vi "take_snapshots_defined_voltage_profile.vi"() -> ()   [LabVIEW 2019]
uses:
  <vilib>/userDefined/High Color/IMAQdx.ctl
  <vilib>/vision/driver/IMAQdx.llb/IMAQdx Attribute Type.ctl
  <vilib>/vision/Management.llb/Cast Image 2 Method.ctl
  <vilib>/DAQmx/write.llb/DAQmx Write (Analog DBL 1Chan 1Samp).vi
  <vilib>/DAQmx/read.llb/DAQmx Read (Analog DBL 1Chan 1Samp).vi
  <vilib>/Analysis/baseanly.llb/Mean (DBL).vi
  <vilib>/DAQmx/create/channels.llb/DAQmx Create Channel (AO-Voltage-Basic).vi
  <vilib>/DAQmx/miscellaneous.llb/DAQmx Fill In Error Info.vi
  <vilib>/DAQmx/create/channels.llb/DAQmx Create Channel (AI-Temperature-Thermocouple).vi
  <vilib>/vision/driver/NI_Vision_Acquisition_Software.lvlib
  <resource>/objmgr/imaqdx.rc
  <vilib>/vision/NI_Vision_Development_Module.lvlib
  <vilib>/Analysis/NI_AALBase.lvlib
  <instrlib>/BK Precision 178XB Series/BK Precision 178XB Series.lvlib
panel:
  out "substring before match":string
  out "number":dbl
  in  "file (use dialog)":path
  in  "DC power supply":refnum<visa-resource-name>="COM3"
  in  "exit PID loop":bool
  in  "Experiment duration\n(min)":dbl
  in  "Snapshot Period\n (min per snapshot)":dbl
  out "Video":bool
  in  "Action":i32(listbox)=1
  out "meanIntensity":dbl[](array[numeric])
  out "varLaplacian":dbl[](array[numeric])
  out "mean":dbl
  out "variance":dbl
  out "Avg Intensity":dbl(graph)=4.716017316017316
  in  "Activate":bool
  out "Var of Laplacian":dbl(graph)=63.940469067936796
  in  "ROI":T1={"Global Rectangle"=[], "Contours"=[{"Contour Type"=0, "ROI Type"=3, "Points"=[231, 86, 235, 90]}, {"Contour Type"=0, "ROI Type"=3, "Points"=[193, 50, 270, 125]}]}
  in  "error in":errorcluster
  in  "File path for video":string="C:\\Users\\Aniket\\Desktop\\mCherry_calibration\\new_lens\\laser_calibration\\laser_and_heating\\"
  in  "Laser profile file path":path=path "C:/Users/Aniket/Desktop/mCherry_calibration/new_lens/laser_calibration/laser_profiles/new_profile.txt"
  in  "Trigger Laser":bool
  in  "Image file path \n(Do not add specify file extension - set to png)":path=path "C:/Users/Aniket/Desktop/mCherry_calibration/new_lens/laser_calibration/laser_profiles.txt"
  out "Current \nTemperature":dbl format="%0.2f"
  out "?":dbl[](graph)=[37.63236695538445]
  out "error out 7":errorcluster
  out "error out 6":errorcluster
  out "error out 5":errorcluster
  out "Exposure Time":dbl
  in  "ON/OFF":bool
  out "error out 3":errorcluster
  in  "LED":dbl(slide) scale=0.0..10.0
  in  "Refresh":bool
  out "Record":bool
  out "Processed Frames per Second":dbl
  out "Acquired Frame Rate":dbl
  out "error out":errorcluster
  out "Camera Display":T2(plugin-control) caption="Image Out"
  in  "Frame Rate":dbl=20.0
  out "Attribute Information Array":T4(array[cluster])
  in  "Session In":T5="cam0"
  # "Camera frame"
  # "Observer frame"
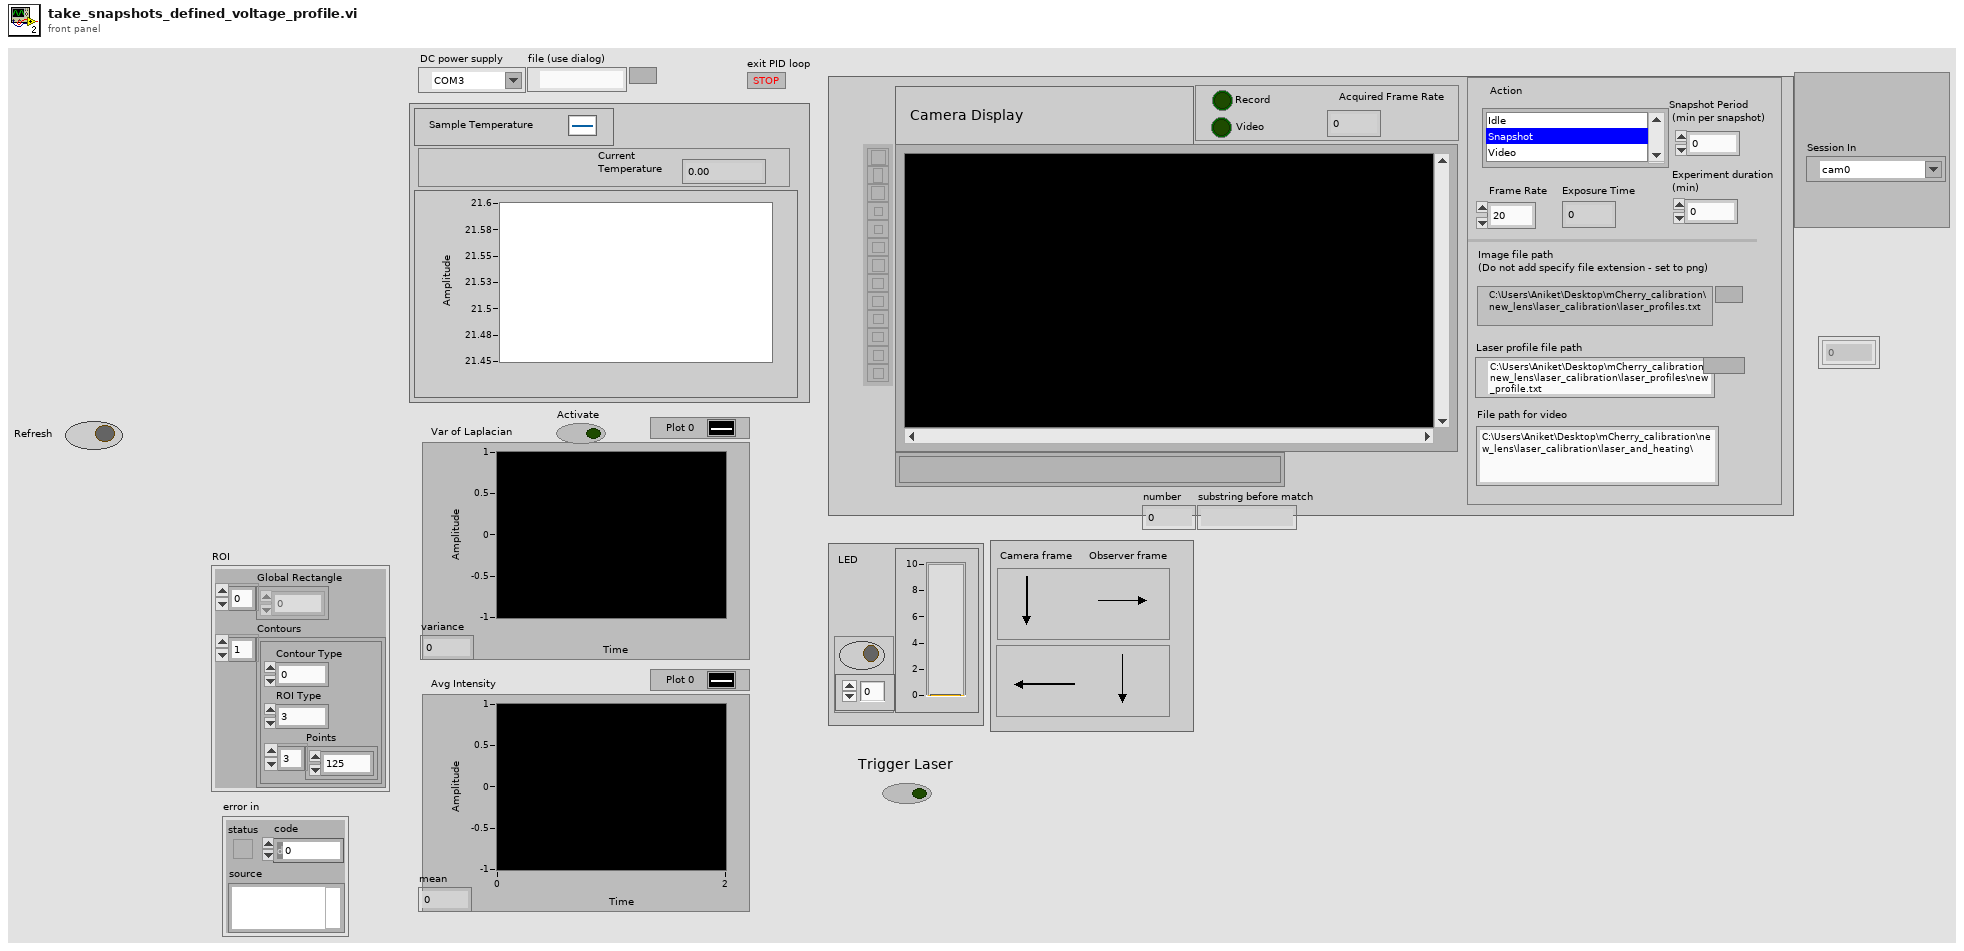
[diagram p1: front panel]
types:
  T1 = cluster{"Global Rectangle":i32[], "Contours":cluster{"Contour Type":u32, "ROI Type":u32, "Points":i32[]}[]}
  T2 = typedef "IMAQ Image.ctl" = refnum<image>
  T3 = typedef "NI_Vision_Acquisition_Software.lvlib/IMAQdx Attribute Type.ctl" = enum32{"U32", "I64", "DBL", "String", "Enum", "Bool", "Command"}
  T4 = cluster{"Attribute Type":T3, "Readable":bool, "Writable":bool, "Attribute Name":string}[]
  T5 = typedef "IMAQdx.ctl" = refnum<k21>
  T6 = typedef "Image Type" = u32
  T7 = typedef "ROI Descriptor" = cluster{"Global Rectangle":i32[], "Contours":cluster{"ID":enum32{"External", "Internal"}, "Type":u32, "Coordinates":i32[]}[]}
  T8 = typedef "IMAQ Rectangle" = cluster{"Left":i32, "Top":i32, "Right":i32, "Bottom":i32, "Rotation":dbl}
  T9 = typedef "Cast Image 2 Method.ctl" = u32
  T10 = typedef "IMAQ AVI2 Refnum.ctl" = refnum<k20>
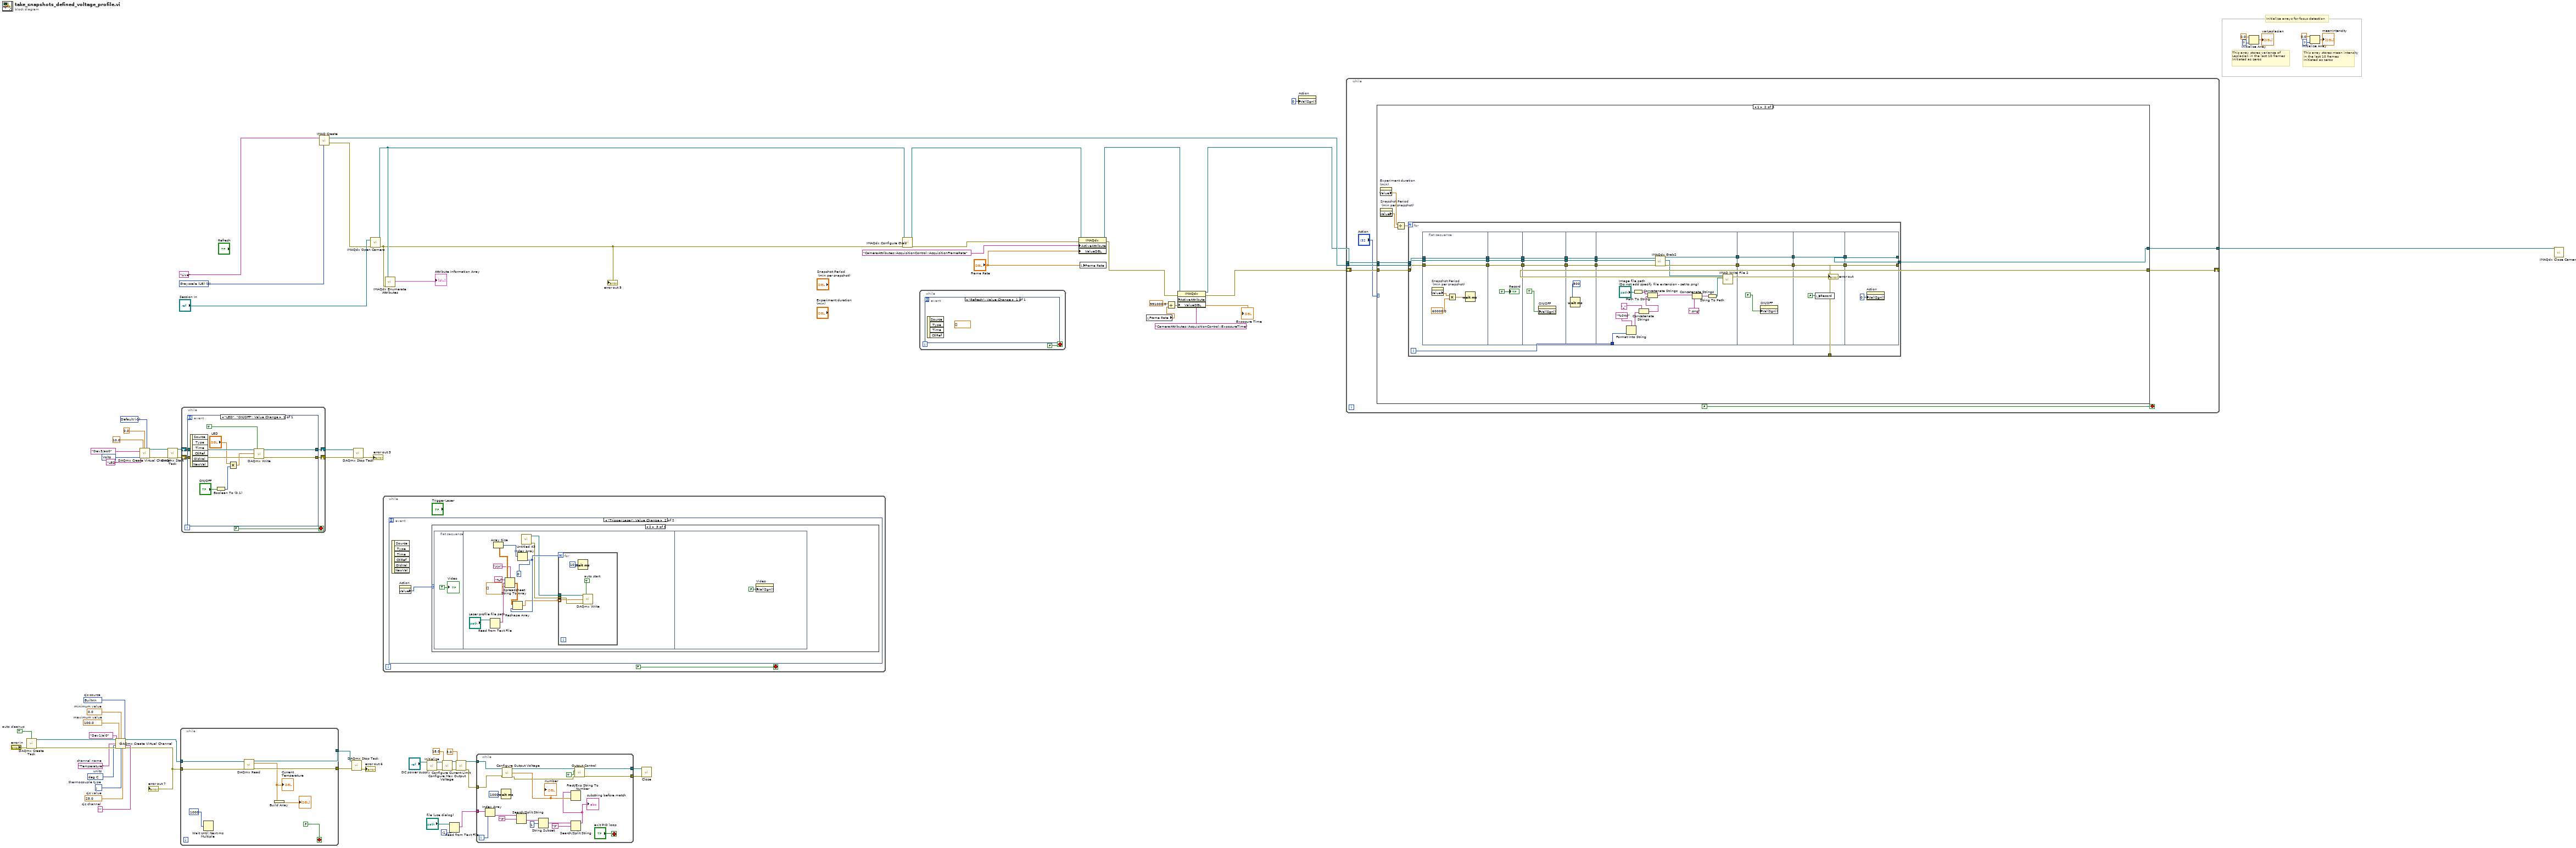
[diagram p0: block diagram]
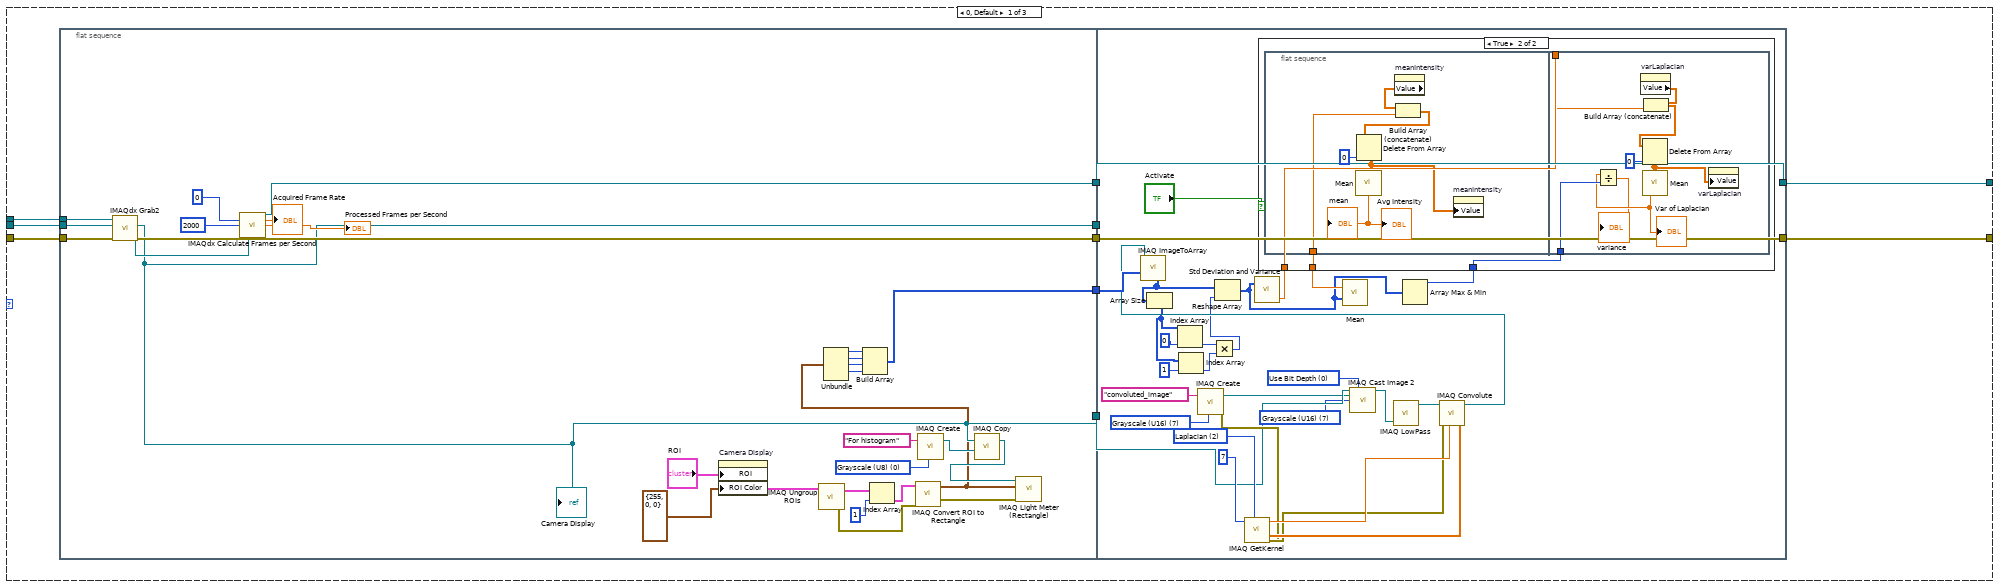
[diagram p2: hidden frame]
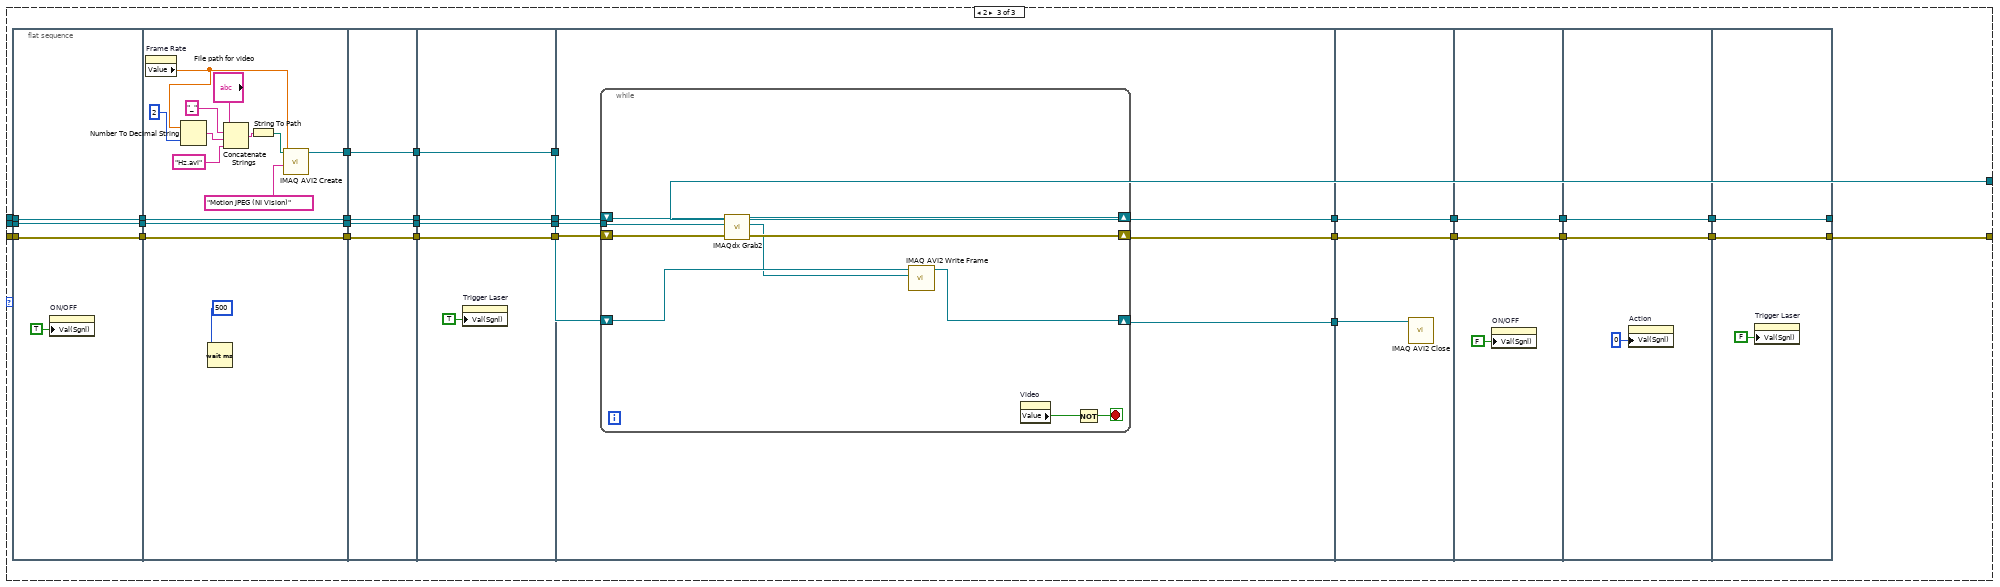
[diagram p4: hidden frame]
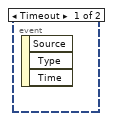
[diagram p5: hidden frame]
diagram:
  w27 = 10200 items=["Built-In"=10200, "Constant Value"=10116, "Channel"=10113]  # cjc source
  w29 = ""  # cjc channel
  w30 = 25.0  # cjc value
  w31 = 10072 items=["J"=10072, "K"=10073, "N"=10077, "R"=10082, "S"=10085, "T"=10086, "B"=10047, "E"=10055]  # thermocouple type
  w32 = 10143 items=["deg C"=10143, "deg F"=10144, "Kelvins"=10325, "deg R"=10145, "From Custom Scale"=10065]  # units
  w28 = "Temperature"  # channel name
  w33 = 0.0  # minimum value
  w34 = 100.0  # maximum value
  w36 = TRUE  # auto cleanup
  w59 = 10348 items=["Volts"=10348, "From Custom Scale"=10065] ("units")
  w61 = -1 items=["Default"=-1, "RSE"=10083, "NRSE"=10078, "Differential"=10106, "Pseudodifferential"=12529] ("input terminal configuration")
  w72 = T6 0 items=["Grayscale (U8)", "Grayscale (I16)", "Grayscale (SGL)", "Complex (CSG)", "RGB (U32)", "HSL (U32)", "RGB (U64)", "Grayscale (U16)"] ("Image Type")
  # "Initialize arrays for focus detection"
  # "This array stores mean intensity in the last 10 frames\nInitiated as zeros"
  # "This array stores variance of Laplacian in the last 10 frames\nInitiated as zeros"
  n1 = call <vilib>:"DAQmx Create Task.vi"("auto cleanup"=w36, "error in"="error in") -> ("task out"=w35:refnum<k21>, "error out"=w37:errorcluster)  [unwired: 12 in]
  n2 = call-poly <vilib>:"DAQmx Create Virtual Channel.vi"("task in"=w35, "maximum value"=w34, "minimum value"=w33, "physical channels"=tag "Dev1/ai0", "cjc source"=w27, "name to assign"=w28, "units"=w32, "cjc channel"=w29, "error in"=w37, "thermocouple type"=w31, "cjc value"=w30) -> ("task out"=w26:refnum<k21>, "error out"=w25:errorcluster)  [unwired: 3 in]
  "error out 7" <- w25
  n3 = call-poly <vilib>:"DAQmx Create Virtual Channel.vi"("maximum value"=10.0, "minimum value"=0.0, "output terminal configuration"=w61, "physical channels"=tag "Dev3/ao0", "name to assign"="LED", "units"=w59) -> ("task out"=w57:refnum<k21>, "error out"=w56:errorcluster)  [unwired: 8 in]
  n4 = call <vilib>:"DAQmx Start Task.vi"("task/channels in"=w57, "error in"=w56) -> ("task out"=w55:refnum<k21>, "error out"=w54:errorcluster)  [unwired: 12 in]
  n5 = while {
    tunnel: w26 -> [w81]
    tunnel: w25 -> [w80]
    tunnel: [w79] -> w41
    tunnel: [w78] -> w40
    stop <- FALSE ("Monitor Temperature") stop-if-true
    n6 = Wait Until Next ms Multiple(millisecond multiple=u32 1000 ("millisecond timer value")) -> ()  [unwired: 1 out]
    n7 = call-poly <vilib>:"DAQmx Read.vi"("task/channels in"=w81, "error in"=w80) -> ("task out"=w79:refnum<k21>, "data"=w75:dbl, "error out"=w78:errorcluster)  [unwired: 11 in]
    "Current \nTemperature" <- w75
    n8 = Build Array(w75) -> (→"?":dbl[])
  }
  n9 = while {
    shift-right: [w85] -> w53
    shift-left: w55 -> [w87]
    shift-right: [w84] -> w52
    shift-left: w54 -> [w86]
    stop <- FALSE stop-if-true
    n10 = event shown="[0] \"LED\", \"ON/OFF\": Value Change" {
      selector: _ -> [_]
      dyn-events: _ -> [_]
      timeout: _ -> [_]
      tunnel: w87 -> [w96]
      tunnel: w86 -> [w95]
      tunnel: [w94] -> w85
      tunnel: [w93] -> w84
      event "LED", "ON/OFF": Value Change {
        n11 = event-data() -> ()  [unwired: 1 in, 6 out]
        n12 = Boolean To (0,1)(Boolean="ON/OFF") -> (0, 1=w89:i16)
        n13 = Multiply(x="LED", y=w89) -> (x*y=w88:dbl)
        n14 = call-poly <vilib>:"DAQmx Write.vi"("task/channels in"=w96, "auto start"=TRUE, "data"=w88, "error in"=w95) -> ("task out"=w94:refnum<k21>, "error out"=w93:errorcluster)  [unwired: 9 in, 1 out]
      }
    }
  }
  n15 = call "IMAQ Create"("Image Name"="Live", "Image Type"=w72) -> ("New Image"=w66:T2, "error out"=w65:errorcluster)  [unwired: 3 in]
  n16 = call <vilib>:"DAQmx Stop Task.vi"("task/channels in"=w41, "error in"=w40) -> ("error out"=→"error out 6":errorcluster)  [unwired: 12 in, 1 out]
  n17 = call <vilib>:"DAQmx Stop Task.vi"("task/channels in"=w53, "error in"=w52) -> ("error out"=→"error out 3":errorcluster)  [unwired: 12 in, 1 out]
  n18 = call <vilib>:"IMAQdx Open Camera.vi"("error in"=w65, "Session In"="Session In") -> ("error out"=w70:errorcluster, "Session Out"=w71:T5)  [unwired: 8 in]
  "error out 5" <- w70
  n19 = while {
    stop <- FALSE stop-if-true
    n20 = event shown="[1] \"Trigger Laser\": Value Change" {
      selector: _ -> [_ _]
      dyn-events: _ -> [_ _]
      timeout: _ -> [_ _]
      event Timeout {
        n21 = event-data() -> ()  [unwired: 1 in, 3 out]
      }
      event "Trigger Laser": Value Change {
        n22 = event-data() -> ()  [unwired: 1 in, 6 out]
        n23 = property on="Action" class="LstBox (strict)"() -> ("Value"=w98:i32)  [unwired: 2 in, 2 out]
        n24 = case shown="2" w98 {
          frame 0, Default {
          }
          frame 1 {
          }
          frame 2 {
            n25 = flat-sequence {
              frame #0 {
                "Video" <- TRUE ("Video")
              }
              frame #1 {
                n26 = Read from Text File(file (use dialog)="Laser profile file path") -> (text=w107:string)  [unwired: 3 in, 3 out]
                n27 = Spreadsheet String To Array(delimiter (Tab)="\r\n", format string="%f", spreadsheet string=w107, array type (2D Dbl)=dbl[][] []) -> (array=w109:dbl[][])
                n28 = Array Size(array=w109) -> (size(s)=w108:i32[])
                n29 = Index Array(array=w108, index=0) -> (element=w111:i32)
                n30 = Reshape Array(w109, w111) -> (w110:dbl[])
                n31 = call "Untitled 43.vi"() -> ("error out"=w100:errorcluster, "task out"=w101:refnum<k21>)  [unwired: 10 in]
                n32 = for {
                  N: w111 -> [_]
                  tunnel: w110 -> [w112] mode=indexing
                  tunnel: w101 -> [w114]
                  tunnel: w100 -> [w113]
                  w115 = TRUE  # auto start
                  n33 = Wait (ms)(milliseconds to wait=u32 10) -> ()  [unwired: 1 out]
                  n34 = call-poly <vilib>:"DAQmx Write.vi"("task/channels in"=w114, "auto start"=w115, "data"=w112, "error in"=w113) -> ()  [unwired: 9 in, 3 out]
                }
              }
              frame #2 {
                n35 = property on="Video" class="Bool (strict)"("Val(Sgnl)"=FALSE ("Value (Signaling)")) -> ()  [unwired: 2 in, 2 out]
              }
            }
          }
        }
      }
    }
  }
  n36 = call <vilib>:"IMAQdx Enumerate Attributes.vi"("error in"=w70, "Session In"=w71) -> ("Attribute Information Array"=→"Attribute Information Array":T4)  [unwired: 7 in, 2 out]
  n37 = call "Initialize.vi"("VISA resource name"="DC power supply") -> ("error out"=w11:errorcluster, "VISA resource name out"=w13:refnum<visa-resource-name>)  [unwired: 9 in]
  n38 = call "Configure Max Output Voltage.vi"("VISA resource name"=w13, "Maximum Output Voltage (18)"=18.0, "error in (no error)"=w11) -> ("VISA resource name out"=w12:refnum<visa-resource-name>, "error out"=w10:errorcluster)  [unwired: 11 in]
  n39 = Read from Text File(file (use dialog)="file (use dialog)", count=-1) -> (text=w7:string[])  [unwired: 2 in, 3 out]
  n40 = call "Configure Current Limit.vi"("VISA resource name"=w12, "Current Limit (0)"=3.0, "error in (no error)"=w10) -> ("VISA resource name out"=w4:refnum<visa-resource-name>, "error out"=w5:errorcluster)  [unwired: 11 in]
  n41 = while {
    tunnel: w7 -> [w135]
    tunnel: [w121] -> w6
    tunnel: w5 -> [w123]
    tunnel: w4 -> [w124]
    tunnel: [w118] -> w3
    i -> [w134]
    stop <- "exit PID loop" stop-if-true
    n42 = Index Array(array=w135, index=w134) -> (element=w133:string)
    n43 = Wait (ms)(milliseconds to wait=u32 1000) -> ()  [unwired: 1 out]
    n44 = Search/Split String(string=w133, search string/char (-)="\t") -> (match + rest of string=w128:string)  [unwired: 1 in, 2 out]
    n45 = String Subset(string=w128, offset (0)=1) -> (substring=w129:string)  [unwired: 1 in]
    n46 = Search/Split String(string=w129, search string/char (-)="\t") -> (substring before match=w126:string)  [unwired: 1 in, 2 out]
    "substring before match" <- w126
    n47 = Fract/Exp String To Number(string=w126) -> (number=w127:dbl)  [unwired: 3 in, 1 out]
    "number" <- w127
    n48 = call "Configure Output Voltage.vi"("VISA resource name"=w124, "Output Voltage (0)"=w127, "error in (no error)"=w123) -> ("VISA resource name out"=w122:refnum<visa-resource-name>, "error out"=w119:errorcluster)  [unwired: 11 in]
    n49 = call "Output Control.vi"("error in (no error)"=w119, "Enable Output Terminals (F: Off)"=TRUE, "VISA resource name"=w122) -> ("error out"=w118:errorcluster, "VISA resource name out"=w121:refnum<visa-resource-name>)  [unwired: 7 in]
  }
  n50 = call "Close.vi"("error in (no error)"=w3, "VISA resource name"=w6) -> ()  [unwired: 9 in, 1 out]
  n51 = call <vilib>:"IMAQdx Configure Grab.vi"("error in"=w70, "Session In"=w71) -> ("error out"=w68:errorcluster, "Session Out"=w50:T5)  [unwired: 8 in]
  n52 = while {
    stop <- FALSE stop-if-true
    n53 = event shown="[0] \"Refresh\": Value Change" {
      selector: _ -> [_]
      dyn-events: _ -> [_]
      timeout: _ -> [_]
      event "Refresh": Value Change {
        (unwired) dbl[] [] ("History Data")
        n54 = event-data() -> ()  [unwired: 1 in, 4 out]
      }
    }
  }
  n55 = property class="IMAQdx"(reference=w50, error in=w68, "ActiveAttribute"="CameraAttributes::AcquisitionControl::AcquisitionFrameRate", "ValueDBL"="Frame Rate") -> (reference out=w45:T5, error out=w43:errorcluster)
  n56 = local write "Frame Rate"("Frame Rate") -> ()
  n57 = local read "Frame Rate"() -> (w47:dbl)
  n58 = Divide(x=991000.0, y=w47) -> (x/y=w46:dbl)
  "Exposure Time" <- w46
  n59 = property class="IMAQdx"(reference=w45, error in=w43, "ActiveAttribute"="CameraAttributes::AcquisitionControl::ExposureTime", "ValueDBL"=w46) -> (reference out=w44:T5, error out=w42:errorcluster)
  n60 = property on="Action" class="LstBox (strict)"("Val(Sgnl)"=0 ("Value (Signaling)")) -> ()  [unwired: 2 in, 2 out]
  n61 = while {
    tunnel: w44 -> [w144]
    tunnel: w66 -> [w142]
    shift-right: [w141] -> w15
    shift-left: w42 -> [w143]
    tunnel: [w138] -> w17
    stop <- FALSE ("Stop") stop-if-true
    n62 = case shown="1" "Action" {
      tunnel: w144 -> [w154 w237 w334]
      tunnel: w143 -> [w153 w235 w332]
      tunnel: w142 -> [w152 w236 w333]
      tunnel: [w151 w234 w330] -> w141
      tunnel: [w150 w233 w331] -> w138
      frame 0, Default {
        n63 = flat-sequence {
          tunnel: w154 -> [w182]
          tunnel: w153 -> [w181]
          tunnel: w152 -> [w180]
          tunnel: [w179] -> w149
          tunnel: [w177] -> w148
          tunnel: [w164] -> w147
          tunnel: [w164] -> w146
          tunnel: [w156] -> w145
          tunnel: [w211] -> w150
          tunnel: [w212] -> w151
          tunnel: w149 -> [w212]
          tunnel: w148 -> [w211]
          tunnel: w147 -> [_]
          tunnel: w146 -> [w192]
          tunnel: w145 -> [w202]
          frame #0 {
            w165 = T6 0 items=["Grayscale (U8)", "Grayscale (I16)", "Grayscale (SGL)", "Complex (CSG)", "RGB (U32)", "HSL (U32)", "RGB (U64)", "Grayscale (U16)"] ("Image Type")
            n64 = call <vilib>:"IMAQdx Grab2.vi"("error in"=w181, "Image In"=w180, "Session In"=w182) -> ("error out"=w179:errorcluster, "Image Out"=w164:T2, "Session Out"=w178:T5)  [unwired: 5 in, 1 out]
            "Camera Display" <- w164
            n65 = call <vilib>:"IMAQdx Calculate Frames per Second.vi"("Session In"=w178, "Buffer Number"=u32 0, "Minimum Display Update Interval (ms)"=u32 2000) -> ("Session Out"=w177:T5, "Acquired Frames per Second"=→"Acquired Frame Rate":dbl, "Processed Frames per Second"=→"Processed Frames per Second":dbl)  [unwired: 6 in, 4 out]
            n66 = property on="Camera Display" class="ImageControl"("ROI"="ROI", "ROI Color"=cluster{"Red":u8, "Green":u8, "Blue":u8} {"Red"=255, "Green"=0, "Blue"=0}) -> ()  [unwired: 2 in, 2 out]
            n67 = call "IMAQ Ungroup ROIs"("ROI Descriptor"="ROI") -> ("error out"=w168:errorcluster, "ROI Descriptors out"=w171:T7[])  [unwired: 3 in]
            n68 = Index Array(array=w171, index=1) -> (element=w169:T7)
            n69 = call "IMAQ Convert ROI to Rectangle"("error in (no error)"=w168, "ROI Descriptor"=w169) -> ("error out"=w167:errorcluster, "Rectangle"=w161:T8)  [unwired: 7 in]
            n70 = Unbundle(w161) -> ("Left"=w160:i32, "Top"=w159:i32, "Right"=w158:i32, "Bottom"=w157:i32)  [unwired: 1 out]
            n71 = Build Array(w160, w159, w158, w157) -> (w156:i32[])
            n72 = call "IMAQ Create"("Image Name"="For histogram", "Image Type"=w165) -> ("New Image"=w163:T2)  [unwired: 3 in, 1 out]
            n73 = call "IMAQ Copy"("Image Dst"=w163, "Image Src"=w164) -> ("Image Dst Out"=w162:T2)  [unwired: 4 in, 1 out]
            n74 = call "IMAQ Light Meter (Rectangle)"("error in (no error)"=w167, "Rectangle"=w161, "Image"=w162) -> ()  [unwired: 4 in, 5 out]
          }
          frame #1 {
            w188 = T6 7 items=["Grayscale (U8)", "Grayscale (I16)", "Grayscale (SGL)", "Complex (CSG)", "RGB (U32)", "HSL (U32)", "RGB (U64)", "Grayscale (U16)"] ("Image Type")
            w191 = T9 0 items=["Use Bit Depth", "Shift", "Use Lookup Table"] ("Method")
            w207 = u16 2 items=["Gradient"=1, "Laplacian"=2, "Smoothing"=3, "Gaussian"=4] ("Kernel Family")
            w209 = T6 7 items=["Grayscale (U8)", "Grayscale (I16)", "Grayscale (SGL)", "Complex (CSG)", "RGB (U32)", "HSL (U32)", "RGB (U64)", "Grayscale (U16)"] ("Image Type")
            n75 = call "IMAQ Create"("Image Name"="convoluted_image", "Image Type"=w209) -> ("New Image"=w190:T2, "error out"=w203:errorcluster)  [unwired: 3 in]
            n76 = call "IMAQ GetKernel"("Kernel Family"=w207, "error in (no error)"=w203, "Kernel Size (3,5,...)"=7) -> ("error out"=w204:errorcluster, "Kernel"=w205:sgl[][], "Divider"=w206:sgl)  [unwired: 5 in, 1 out]
            n77 = call "IMAQ Cast Image 2"("Image Src"=w192, "Method"=w191, "Image Dst"=w190, "Image Type"=w188) -> ("Image Dst Out"=w189:T2)  [unwired: 10 in, 1 out]
            n78 = call "IMAQ LowPass"("Image Src"=w189) -> ("Image Dst Out"=w193:T2)  [unwired: 6 in, 1 out]
            n79 = call "IMAQ Convolute"("Kernel"=w205, "Divider (kernel sum)"=w206, "error in (no error)"=w204, "Image Src"=w193) -> ("Image Dst Out"=w201:T2)  [unwired: 6 in, 1 out]
            n80 = call "IMAQ ImageToArray"("Optional Rectangle"=w202, "Image"=w201) -> ("Image Pixels (U16)"=w186:u16[][])  [unwired: 2 in, 4 out]
            n81 = Array Size(array=w186) -> (size(s)=w187:i32[])
            n82 = Index Array(array=w187, index=0 ("index (row)")) -> (element=w198:i32)
            n83 = Index Array(array=w187, index=1) -> (element=w197:i32)
            n84 = Multiply(x=w198, y=w197) -> (x*y=w185:i32)
            n85 = Reshape Array(w186, w185) -> (w184:u16[])
            n86 = call <vilib>:"Std Deviation and Variance.vi"("X"=w184) -> ("variance"=w195:dbl)  [unwired: 1 in, 2 out]
            n87 = call-poly <vilib>:"Mean.vi"("X"=w184) -> ("mean"=w194:dbl)  [unwired: 1 out]
            n88 = Array Max & Min(array=w184) -> (max value=w183:u16)  [unwired: 3 out]
            n89 = case shown="True" "Activate" {
              tunnel: w195 -> [_ w214]
              tunnel: w194 -> [_ w215]
              tunnel: w183 -> [_ w213]
              frame False {
              }
              frame True {
                n90 = flat-sequence {
                  tunnel: w215 -> [w218]
                  tunnel: w214 -> [w224]
                  tunnel: w213 -> [w229]
                  frame #0 {
                    n91 = property on="meanIntensity" class="Arr (strict)"() -> ("Value"=w219:dbl[])  [unwired: 2 in, 2 out]
                    n92 = Build Array (concatenate)(w219, w218) -> (w217:dbl[])
                    n93 = Delete From Array(array=w217, index=0) -> (array with subset deleted=w216:dbl[])  [unwired: 1 in, 1 out]
                    n94 = call-poly <vilib>:"Mean.vi"("X"=w216) -> ("mean"=→"Avg Intensity" →"mean":dbl)  [unwired: 1 out]
                    n95 = property on="meanIntensity" class="Arr (strict)"("Value"=w216) -> ()  [unwired: 2 in, 2 out]
                  }
                  frame #1 {
                    n96 = property on="varLaplacian" class="Arr (strict)"() -> ("Value"=w225:dbl[])  [unwired: 2 in, 2 out]
                    n97 = Build Array (concatenate)(w225, w224) -> (w223:dbl[])
                    n98 = Delete From Array(array=w223, index=0) -> (array with subset deleted=w222:dbl[])  [unwired: 1 in, 1 out]
                    n99 = call-poly <vilib>:"Mean.vi"("X"=w222) -> ("mean"=w228:dbl)  [unwired: 1 out]
                    "Var of Laplacian" <- w228
                    n100 = Divide(x=w228, y=w229) -> (x/y=→"variance":dbl)
                    n101 = property on="varLaplacian" class="Arr (strict)"("Value"=w222) -> ()  [unwired: 2 in, 2 out]
                  }
                }
              }
            }
          }
        }
      }
      frame 1 {
        n102 = property on="Experiment duration\n(min)" class="DigNum (strict)"() -> ("Value"=w231:dbl)  [unwired: 2 in, 2 out]
        n103 = property on="Snapshot Period\n (min per snapshot)" class="DigNum (strict)"() -> ("Value"=w230:dbl)  [unwired: 2 in, 2 out]
        n104 = Divide(x=w231, y=w230) -> (x/y=w232:dbl)
        n105 = for {
          N: w232 -> [_]
          tunnel: w237 -> [w246]
          tunnel: w236 -> [w245]
          tunnel: w235 -> [w244]
          tunnel: [w243] -> w234
          tunnel: [w242] -> w233
          i -> [w241]
          n106 = flat-sequence {
            tunnel: w246 -> [w265]
            tunnel: w245 -> [w266]
            tunnel: w244 -> [w267]
            tunnel: [w267] -> w240
            tunnel: [w266] -> w239
            tunnel: [w265] -> w238
            tunnel: [w271] -> w261
            tunnel: [w270] -> w260
            tunnel: [w269] -> w259
            tunnel: w238 -> [w269]
            tunnel: w239 -> [w270]
            tunnel: w240 -> [w271]
            tunnel: [w275] -> w258
            tunnel: [w274] -> w257
            tunnel: [w273] -> w256
            tunnel: w261 -> [w275]
            tunnel: w260 -> [w274]
            tunnel: w259 -> [w273]
            tunnel: w258 -> [w279]
            tunnel: [w279] -> w255
            tunnel: w257 -> [w278]
            tunnel: [w278] -> w254
            tunnel: w256 -> [w277]
            tunnel: [w277] -> w253
            tunnel: [w292] -> w252
            tunnel: [w296] -> w251
            tunnel: w255 -> [w295]
            tunnel: w254 -> [w294]
            tunnel: w253 -> [w293]
            tunnel: w241 -> [w280]
            tunnel: w252 -> [w299]
            tunnel: [w299] -> w250
            tunnel: w251 -> [w298]
            tunnel: [w298] -> w249
            tunnel: w250 -> [w302]
            tunnel: w249 -> [w301]
            tunnel: [w302] -> w248
            tunnel: [w301] -> w247
            tunnel: [w305] -> w243
            tunnel: [w303] -> w242
            tunnel: w248 -> [w303]
            tunnel: w247 -> [w305]
            frame #0 {
              n107 = property on="Snapshot Period\n (min per snapshot)" class="DigNum (strict)"() -> ("Value"=w264:dbl)  [unwired: 2 in, 2 out]
              n108 = Multiply(x=w264, y=60000.0) -> (x*y=w262:dbl)
              n109 = Wait (ms)(milliseconds to wait=w262) -> ()  [unwired: 1 out]
            }
            frame #1 {
              "Record" <- TRUE ("Record")
            }
            frame #2 {
              n110 = property on="ON/OFF" class="Bool (strict)"("Val(Sgnl)"=TRUE ("ON/OFF")) -> ()  [unwired: 2 in, 2 out]
            }
            frame #3 {
              n111 = Wait (ms)(milliseconds to wait=u32 500) -> ()  [unwired: 1 out]
            }
            frame #4 {
              n112 = Format Into String(format string="%04d", w280) -> (resulting string=w281:string)  [unwired: 2 in, 1 out]
              n113 = Path To String(path="Image file path \n(Do not add specify file extension - set to png)") -> (string=w288:string)
              n114 = Concatenate Strings("_" ("string"), w281) -> (w287:string)
              n115 = Concatenate Strings(w288, w287) -> (w286:string)
              n116 = call <vilib>:"IMAQdx Grab2.vi"("error in"=w295, "Image In"=w294, "Session In"=w293) -> ("error out"=w296:errorcluster, "Image Out"=w291:T2, "Session Out"=w292:T5)  [unwired: 5 in, 1 out]
              n117 = Concatenate Strings(w286, ".png" ("string")) -> (w284:string)
              n118 = String To Path(string=w284) -> (path=w283:path)
              n119 = call-poly "IMAQ Write File 2"("File Path"=w283, "Image"=w291) -> ()  [unwired: 8 in, 2 out]
            }
            frame #5 {
              n120 = property on="ON/OFF" class="Bool (strict)"("Val(Sgnl)"=FALSE ("ON/OFF")) -> ()  [unwired: 2 in, 2 out]
            }
            frame #6 {
              n121 = local write "Record"(FALSE ("Record")) -> ()
            }
            frame #7 {
              n122 = property on="Action" class="LstBox (strict)"("Val(Sgnl)"=0 ("Value (Signaling)")) -> ()  [unwired: 2 in, 2 out]
            }
          }
        }
      }
      frame 2 {
        n123 = flat-sequence {
          tunnel: w332 -> [w336]
          tunnel: w333 -> [w337]
          tunnel: w334 -> [w338]
          tunnel: [w338] -> w329
          tunnel: [w337] -> w328
          tunnel: [w336] -> w327
          tunnel: w329 -> [w352]
          tunnel: [w352] -> w326
          tunnel: w328 -> [w351]
          tunnel: [w351] -> w324
          tunnel: w327 -> [w350]
          tunnel: [w350] -> w322
          tunnel: [w347] -> w315
          tunnel: w326 -> [w356]
          tunnel: [w356] -> w325
          tunnel: w324 -> [w355]
          tunnel: [w355] -> w323
          tunnel: w322 -> [w354]
          tunnel: [w354] -> w321
          tunnel: [w353] -> w316
          tunnel: w315 -> [w353]
          tunnel: w325 -> [w358]
          tunnel: w323 -> [w359]
          tunnel: w321 -> [w360]
          tunnel: [w360] -> w320
          tunnel: [w359] -> w319
          tunnel: [w358] -> w318
          tunnel: [w357] -> w317
          tunnel: w316 -> [w357]
          tunnel: w320 -> [w367]
          tunnel: w319 -> [w366]
          tunnel: w318 -> [w365]
          tunnel: [w363] -> w314
          tunnel: [w364] -> w313
          tunnel: [w368] -> w312
          tunnel: w317 -> [w362]
          tunnel: w314 -> [w381]
          tunnel: [w381] -> w309
          tunnel: w313 -> [w380]
          tunnel: [w380] -> w311
          tunnel: w312 -> [w379]
          tunnel: w311 -> [w384]
          tunnel: [w384] -> w310
          tunnel: w309 -> [w383]
          tunnel: [w383] -> w308
          tunnel: w310 -> [w386]
          tunnel: w308 -> [w387]
          tunnel: [w387] -> w307
          tunnel: [w386] -> w306
          tunnel: [w389] -> w330
          tunnel: [w390] -> w331
          tunnel: w307 -> [w390]
          tunnel: w306 -> [w389]
          frame #0 {
            n124 = property on="ON/OFF" class="Bool (strict)"("Val(Sgnl)"=TRUE ("Value (Signaling)")) -> ()  [unwired: 2 in, 2 out]
          }
          frame #1 {
            n125 = property on="Frame Rate" class="DigNum (strict)"() -> ("Value"=w345:dbl)  [unwired: 2 in, 2 out]
            n126 = Number To Decimal String(number=w345, width (-)=i16 2) -> (decimal integer string=w340:string)
            n127 = Wait (ms)(milliseconds to wait=u32 500) -> ()  [unwired: 1 out]
            n128 = Concatenate Strings("File path for video", "_" ("string"), w340, "Hz.avi" ("string")) -> (w342:string)
            n129 = String To Path(string=w342) -> (path=w343:path)
            n130 = call "IMAQ AVI2 Create"("Codec"="Motion JPEG (NI Vision)", "Frames Per Second"=w345, "AVI Path"=w343) -> ("AVI Refnum"=w347:T10)  [unwired: 7 in, 1 out]
          }
          frame #2 {
          }
          frame #3 {
            n131 = property on="Trigger Laser" class="Bool (strict)"("Val(Sgnl)"=TRUE ("Value (Signaling)")) -> ()  [unwired: 2 in, 2 out]
          }
          frame #4 {
            n132 = while {
              tunnel: w366 -> [w376]
              shift-right: [w374] -> w364
              shift-left: w367 -> [w377]
              shift-right: [w373] -> w363
              shift-left: w365 -> [w375]
              shift-right: [w378] -> w368
              shift-left: w362 -> [w372]
              stop <- w370 stop-if-true
              n133 = call <vilib>:"IMAQdx Grab2.vi"("error in"=w377, "Image In"=w376, "Session In"=w375) -> ("error out"=w374:errorcluster, "Image Out"=w371:T2, "Session Out"=w373:T5)  [unwired: 5 in, 1 out]
              n134 = call "IMAQ AVI2 Write Frame"("Image"=w371, "AVI Refnum"=w372) -> ("AVI Refnum (duplicate)"=w378:T10)  [unwired: 7 in, 2 out]
              n135 = property on="Video" class="Bool (strict)"() -> ("Value"=w369:bool)  [unwired: 2 in, 2 out]
              n136 = Not(x=w369) -> (.not. x?=w370:bool)
            }
          }
          frame #5 {
            n137 = call "IMAQ AVI2 Close"("AVI Refnum"=w379) -> ()  [unwired: 10 in, 1 out]
          }
          frame #6 {
            n138 = property on="ON/OFF" class="Bool (strict)"("Val(Sgnl)"=FALSE ("Value (Signaling)")) -> ()  [unwired: 2 in, 2 out]
          }
          frame #7 {
            n139 = property on="Action" class="LstBox (strict)"("Val(Sgnl)"=0 ("Value (Signaling)")) -> ()  [unwired: 2 in, 2 out]
          }
          frame #8 {
            n140 = property on="Trigger Laser" class="Bool (strict)"("Val(Sgnl)"=FALSE ("Value (Signaling)")) -> ()  [unwired: 2 in, 2 out]
          }
        }
      }
    }
  }
  "error out" <- w15
  n141 = Initialize Array(0.0 ("element"), 7 ("dimension size")) -> (→"varLaplacian":dbl[])
  n142 = Initialize Array(0.0 ("element"), 7 ("dimension size")) -> (→"meanIntensity":dbl[])
  n143 = call <vilib>:"IMAQdx Close Camera.vi"("Session In"=w17) -> ()  [unwired: 10 in, 1 out]
